vi "array -- interpolate -- i.vi"(4 "all Voltage":dbl[](array[numeric]), 6 "all tempearure":dbl[](array[numeric]), 8 "weights":dbl[](array[numeric]), 11 "temperature (K)":dbl) -> (2 "V out":dbl=0.01)   [LabVIEW 2015]
uses:
  Q - not nan -- real.vi
  <vilib>/gmath/NI_Gmath.lvlib
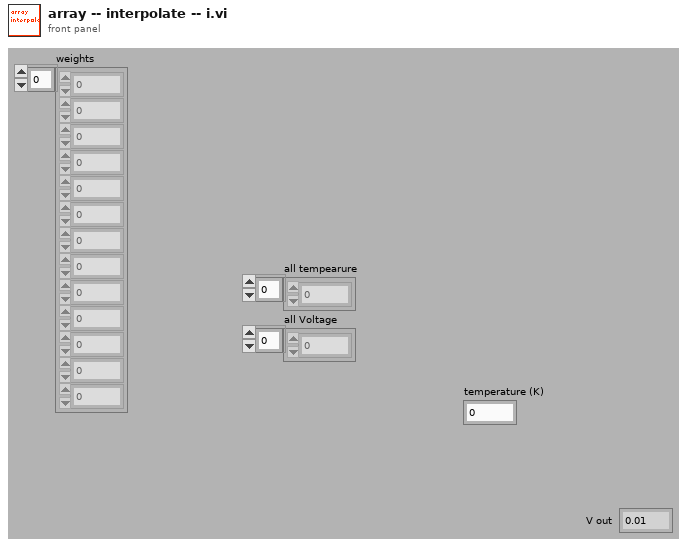
[diagram p1: front panel]
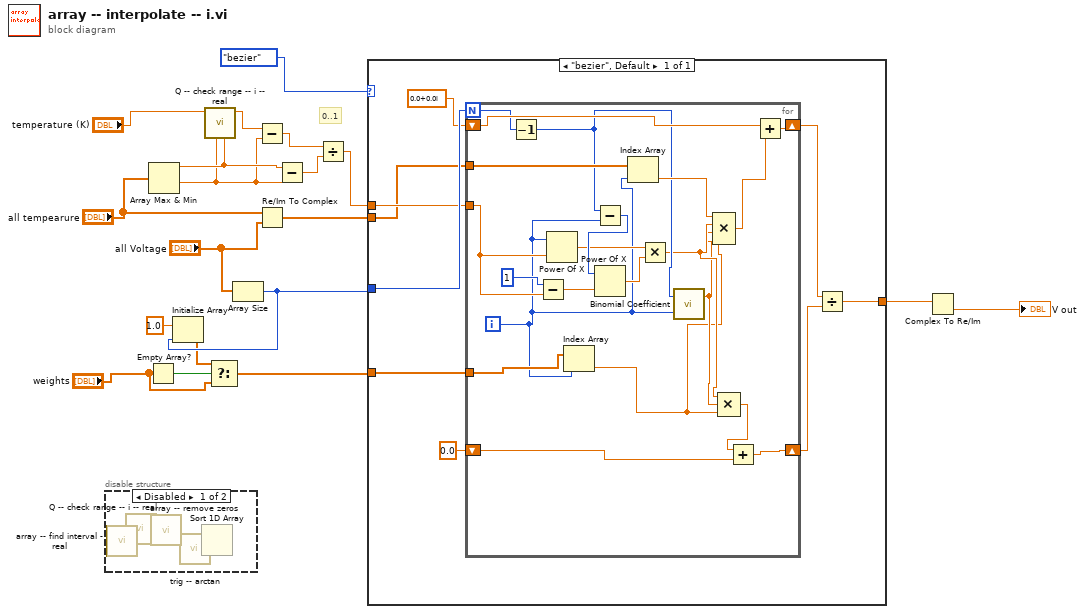
[diagram p0: block diagram]
diagram:
  # "0..1"
  n1 = disable-structure shown="Disabled" {
    frame Disabled {
      n2 = call "array -- find interval - real.vi"() -> ("number"=w20:dbl)  [unwired: 5 in, 6 out]
      n3 = call "Q -- check range -- i -- real.vi"() -> ()  [unwired: 9 in, 3 out]
      n4 = call "array -- remove zeros.vi"() -> ()  [unwired: 11 in, 1 out]
      n5 = call "trig -- arctan.vi"() -> ()  [unwired: 15 in, 1 out]
      n6 = Sort 1D Array() -> ()  [unwired: 1 in, 1 out]
    }
    frame Enabled {
    }
  }
  n7 = Empty Array?(array="weights") -> (empty?=w6:bool)
  n8 = Array Max & Min(array="all tempearure") -> (max value=w15:dbl, min value=w14:dbl)  [unwired: 2 out]
  n9 = call "Q -- check range -- i -- real.vi"("upper"=w15, "lower"=w14, "number"="temperature (K)") -> ("number in range"=w16:dbl)  [unwired: 6 in, 2 out]
  n10 = Array Size(array="all Voltage") -> (size(s)=w4:i32)
  n11 = Initialize Array(1.0 ("element"), w4) -> (w3:dbl[])
  n12 = Select(t=w3, s=w6, f="weights") -> (s? t:f=w1:dbl[])
  n13 = Subtract(x=w16, y=w14) -> (x-y=w12:dbl)
  n14 = Re/Im To Complex(1:"all Voltage", 2:"all tempearure") -> (0:w9:cdb[])
  n15 = Subtract(x=w15, y=w14) -> (x-y=w13:dbl)
  n16 = Divide(x=w12, y=w13) -> (x/y=w10:dbl)
  n17 = case shown="\"bezier\", Default" enum16{"bezier", "other"}."bezier" {
    tunnel: w4 -> [w29]
    tunnel: w10 -> [w28]
    tunnel: w9 -> [w27]
    tunnel: [w21] -> w8
    tunnel: w1 -> [w25]
    frame "bezier", Default {
      n18 = for {
        N: w29 -> [w39]
        tunnel: w28 -> [w49]
        tunnel: w27 -> [w44]
        shift-right: [w40] -> w23
        shift-left: cdb 0.0+0.0i -> [w42]
        tunnel: w25 -> [w35]
        shift-right: [w33] -> w22
        shift-left: 0.0 -> [w31]
        i -> [w34]
        n19 = Decrement(x=w39) -> (x-1=w38:i32)
        n20 = Subtract(x=1, y=w49) -> (x-y=w48:dbl)
        n21 = Power Of X(1:w49, 2:w34) -> (0:w46:dbl)
        n22 = Index Array(array=w35, index=w34) -> (element=w30:dbl)
        n23 = Subtract(x=w38, y=w34) -> (x-y=w47:i32)
        n24 = Power Of X(1:w48, 2:w47) -> (0:w45:dbl)
        n25 = Index Array(array=w44, index=w34) -> (element=w43:cdb)
        n26 = Multiply(x=w46, y=w45) -> (x*y=w37:dbl)
        n27 = call <vilib>:"Binomial Coefficient.vi"("k"=w34, "n"=w38) -> ("binomial coefficient (n,k)"=w36:dbl)  [unwired: 1 out]
        n28 = Compound Arithmetic op=MULTIPLY(w43, w37, w36, w30) -> (w41:cdb)
        n29 = Compound Arithmetic op=MULTIPLY(w37, w36, w30) -> (w32:dbl)
        n30 = Add(x=w32, y=w31) -> (x+y=w33:dbl)
        n31 = Add(x=w42, y=w41) -> (x+y=w40:cdb)
      }
      n32 = Divide(x=w23, y=w22) -> (x/y=w21:cdb)
    }
  }
  n33 = Complex To Re/Im(x + iy=w8) -> (y=→"V out":dbl)  [unwired: 1 out]
